vi "libssh2_channel_window_write_ex.vi"(8 "error in (no error)":errorcluster, 11 "channel":T1) -> (0 "error out":errorcluster, 2 "initial window size":u32, 3 "remaining write window":u32)   [LabVIEW 2013, in "libssh2.lvlib"]
doc: "Returns the number of bytes which may safely be written on the channel without blocking.\n\n<B>initial window size</B> returns the initial window size as defined by the channel_open request. It may be zero for locally initiated channels."
uses:
  libssh2.lvlib
  Channel Refnum.ctl
  Not A Channel.vi
  <vilib>/Utility/error.llb/Error Cluster From Error Code.vi
  Global Settings.vi
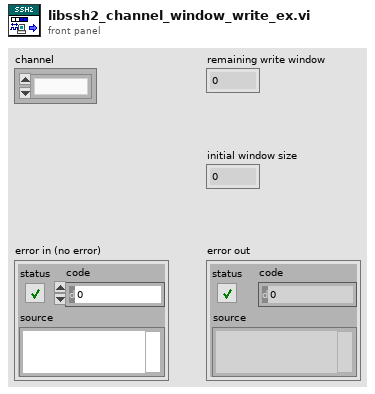
[diagram p1: front panel]
types:
  T1 = typedef "libssh2.lvlib/Channel Refnum.ctl" = refnum<k1>
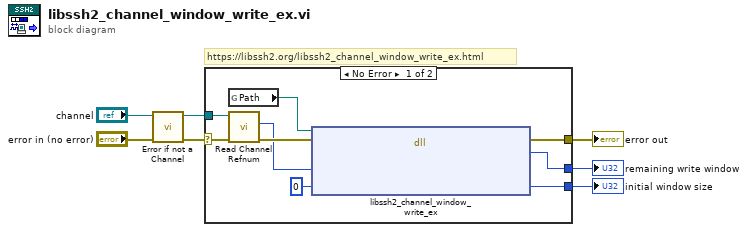
[diagram p0: block diagram]
diagram:
  # "https://libssh2.org/libssh2_channel_window_write_ex.html"
  n1 = call "Error if not a Channel.vi"("error in (no error)"="error in (no error)", "channel"="channel") -> ("error out"=w3:errorcluster, "channel out"=w1:T1)  [unwired: 8 in]
  n2 = case shown="No Error" w3 {
    selector: w3 -> [w16 w17]
    tunnel: [w15 w17] -> w7
    tunnel: w1 -> [w14 _]
    tunnel: [w13 _] -> w5
    tunnel: [w12 _] -> w4
    frame No Error {
      n3 = global read "Global Settings.vi" "Path"() -> (w9:path)
      n4 = call "Read Channel Refnum.vi"("error in (no error)"=w16, "channel"=w14) -> ("error out"=w11:errorcluster, "LIBSSH2_CHANNEL*"=w10:u64)  [unwired: 8 in]
      n5 = dll-call lib="?" fn="libssh2_channel_window_write_ex"(path in=w9, error in=w11, "channel"=w10, "window_size_initial"=u32 0) -> (error out=w15:errorcluster, "return value"=w12:u32, "window_size_initial"=w13:u32)  [unwired: 2 in, 1 out]
    }
    frame Error {
    }
  }
  "error out" <- w7
  "initial window size" <- w5
  "remaining write window" <- w4
